vi "RFH-save-common_format.vi"(7 "file path (use dialog)":path, 8 "error in (no error)":errorcluster, 10 "Common Format":T1) -> (0 "error out":errorcluster)   [LabVIEW 2020, in "RFH-Reflection_File_Handler.lvlib"]
uses:
  RFH-Reflection_File_Handler.lvlib
  RFH-common_data_format.ctl
  <vilib>/Utility/file.llb/Write Delimited Spreadsheet (DBL).vi
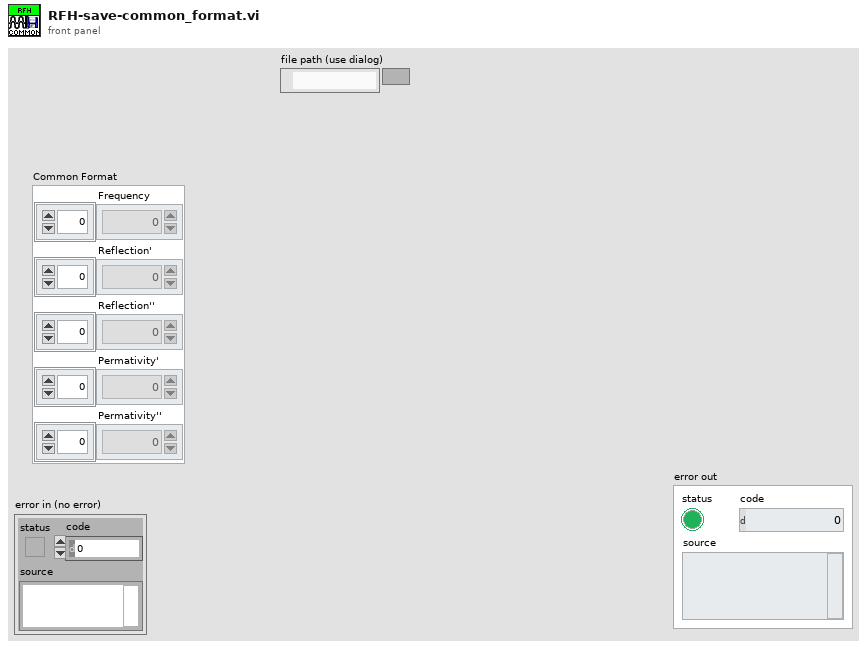
[diagram p1: front panel]
types:
  T1 = typedef "RFH-Reflection_File_Handler.lvlib/RFH-common_data_format.ctl" = cluster{"Frequency":dbl[], "Reflection'":dbl[], "Reflection''":dbl[], "Permativity'":dbl[], "Permativity''":dbl[]}
  T2 = enum16{"open", "replace", "create", "open or create", "replace or create", "replace or create with confirmation"}
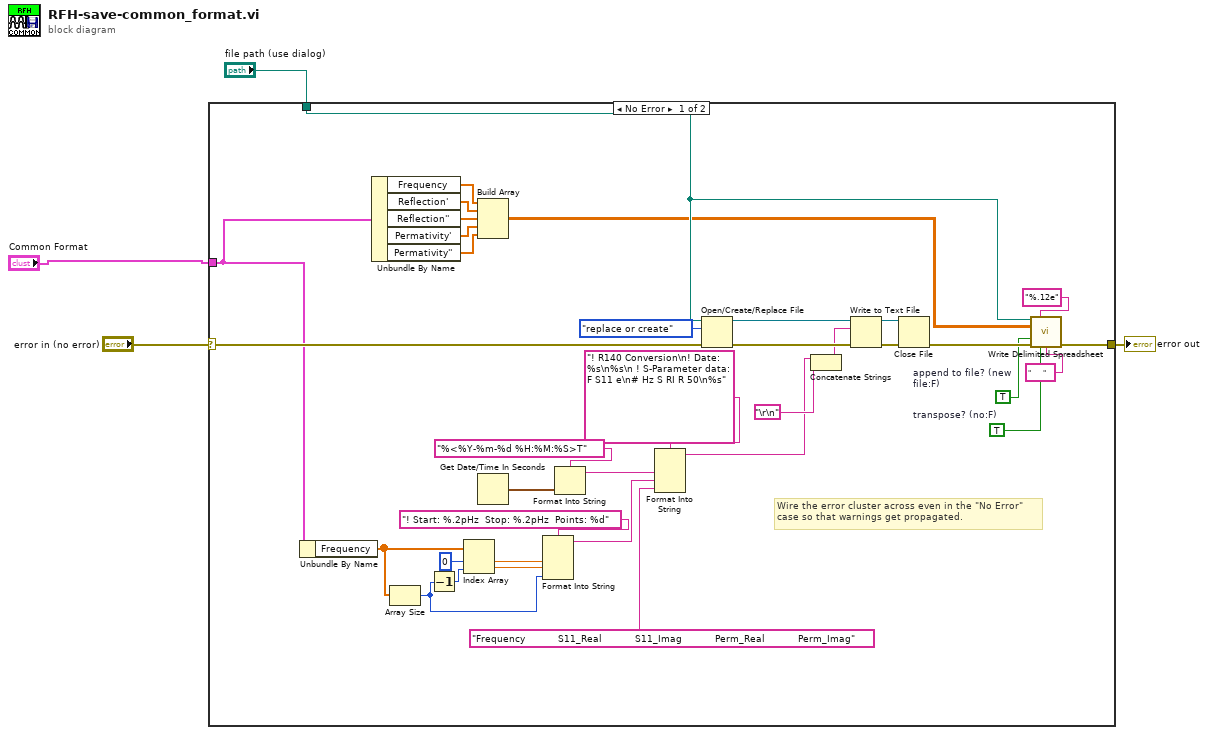
[diagram p0: block diagram]
diagram:
  n1 = case shown="No Error" "error in (no error)" {
    selector: "error in (no error)" -> [w13 w41]
    tunnel: [w5 w41] -> w2
    tunnel: "Common Format" -> [w6 _]
    tunnel: "file path (use dialog)" -> [w20 _]
    frame No Error {
      w22 = TRUE  # append to file? (new file:F)
      w24 = TRUE  # transpose? (no:F)
      # "Wire the error cluster across even in the \"No Error\"\ncase so that warnings get propagated."
      n2 = Unbundle By Name(w6) -> ("Frequency"=w12:dbl[])
      n3 = Unbundle By Name(w6) -> ("Frequency"=w17:dbl[], "Reflection'"=w19:dbl[], "Reflection''"=w18:dbl[], "Permativity'"=w16:dbl[], "Permativity''"=w15:dbl[])
      n4 = Array Size(array=w12) -> (size(s)=w7:i32)
      n5 = Decrement(x=w7) -> (x-1=w11:i32)
      n6 = Index Array(array=w12, index #1=0 ("index"), index #2=w11) -> (element #1=w9:dbl, element #2=w8:dbl)
      n7 = Build Array(w17, w19, w18, w16, w15) -> (w14:dbl[][])
      n8 = Get Date/Time In Seconds() -> (seconds since 1Jan1904=w31:timestamp)
      n9 = Format Into String(format string="! Start: %.2pHz  Stop: %.2pHz  Points: %d", w9, w8, w7) -> (resulting string=w27:string)  [unwired: 2 in, 1 out]
      n10 = Format Into String(format string="%<%Y-%m-%d %H:%M:%S>T", w31) -> (resulting string=w29:string)  [unwired: 2 in, 1 out]
      n11 = Format Into String(format string="! R140 Conversion\n! Date: %s\n%s\n ! S-Parameter data: F S11 e\n# Hz S RI R 50\n%s" ("text"), w29, w27, "Frequency           S11_Real           S11_Imag           Perm_Real           Perm_Imag" ("input 3")) -> (resulting string=w33:string)  [unwired: 2 in, 1 out]
      n12 = Open/Create/Replace File(file path (use dialog)=w20, error in=w13, operation (0:open)=T2."replace or create") -> (refnum out=w37:refnum<file>, error out=w38:errorcluster)  [unwired: 3 in, 1 out]
      n13 = Concatenate Strings(w33, "\r\n") -> (w34:string)
      n14 = Write to Text File(file (use dialog)=w37, text=w34, error in=w38) -> (refnum out=w39:refnum<file>, error out=w40:errorcluster)  [unwired: 1 in, 1 out]
      n15 = Close File(refnum=w39, error in=w40) -> (error out=w23:errorcluster)  [unwired: 1 out]
      n16 = call-poly <vilib>:"Write Delimited Spreadsheet.vi"("file path (dialog if empty)"=w20, "format (%.3f)"="%.12e", "2D data"=w14, "append to file? (new file:F)"=w22, "error in (no error)"=w23, "transpose? (no:F)"=w24, "delimiter (\\t)"="      " ("delimiter (\\t)")) -> ("error out"=w5:errorcluster)  [unwired: 7 in, 1 out]
    }
    frame Error {
    }
  }
  "error out" <- w2
